vi "arbitrary_stimulus.vi"(8 "index":i32, 10 "Set signal":bool, 11 "New signal":sgl[][](array[numeric])) -> (1 "Value":sgl[](array[numeric]), 3 "Length":i32)   [LabVIEW 2013]
panel:
  # "This is a functional array variable used to avoid copying the stimulus array.  \nDon't call this directly to set the stimulus, use set_arbitrary_stimulus."
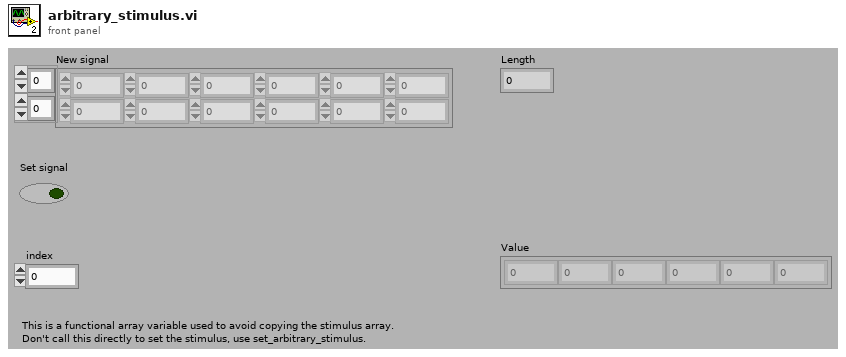
[diagram p1: front panel]
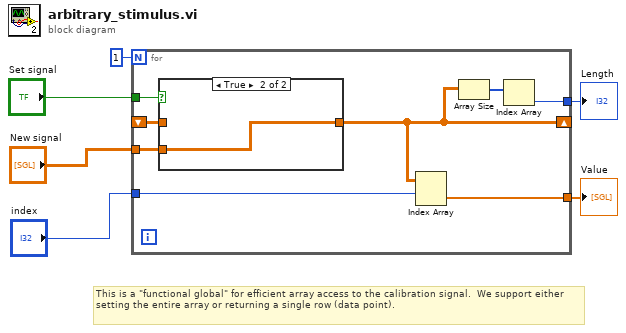
[diagram p0: block diagram]
diagram:
  # "This is a \"functional global\" for efficient array access to the calibration signal.  We support either setting the entire array or returning a single row (data point)."
  n1 = for {
    N: 1 -> [_]
    shift-right: [w9] -> _
    shift-left: _ -> [w12]
    tunnel: "Set signal" -> [w14]
    tunnel: "New signal" -> [w13]
    tunnel: "index" -> [w11]
    tunnel: [w10] -> w2
    tunnel: [w7] -> w1
    n2 = case shown="True" w14 {
      tunnel: w13 -> [_ w16]
      tunnel: [w15 w16] -> w9
      tunnel: w12 -> [w15 _]
      frame False {
      }
      frame True {
      }
    }
    n3 = Index Array(array=w9, index (row)=w11) -> (element=w10:sgl[])  [unwired: 1 in]
    n4 = Array Size(array=w9) -> (size(s)=w8:i32[])
    n5 = Index Array(array=w8) -> (element=w7:i32)  [unwired: 1 in]
  }
  "Value" <- w2
  "Length" <- w1
